vi "arrange pamameter.vi"(1 "meaSetId(SA)":i32[](array[numeric]), 2 "meaSetId(Volt)":i32[](array[numeric])) -> (0 "Arrange MeasSetid":i32[](array[numeric]))   [LabVIEW 2016]
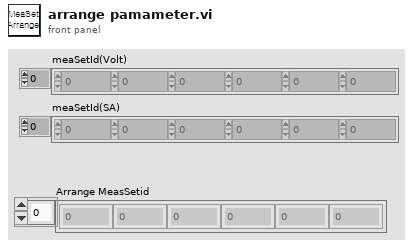
[diagram p1: front panel]
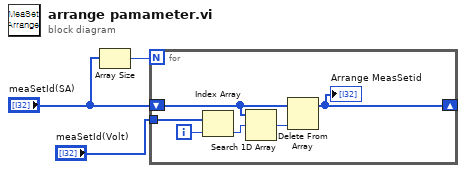
[diagram p0: block diagram]
diagram:
  n1 = Array Size(array="meaSetId(SA)") -> (size(s)=w3:i32)
  n2 = for {
    N: w3 -> [_]
    tunnel: "meaSetId(Volt)" -> [w9]
    shift-right: [w4] -> _
    shift-left: "meaSetId(SA)" -> [w6]
    i -> [w8]
    n3 = Index Array(array=w9, index=w8) -> (element=w7:i32)
    n4 = Search 1D Array(1D array=w6, element=w7) -> (index of element=w5:i32)  [unwired: 1 in]
    n5 = Delete From Array(array=w6, index=w5) -> (array with subset deleted=w4:i32[])  [unwired: 1 in, 1 out]
    "Arrange MeasSetid" <- w4
  }
